vi "SMO_Query.vi"(0 "System no.":i32=1 min=1 max=4 step=1, 2 "Axes to query":string[](array[string]), 3 "All axes?":bool, 4 "Axis identifier?":bool=TRUE, 5 "error in":errorcluster) -> (14 "Current motor output":dbl[](array[numeric]) format="%.6f", 19 "error out":errorcluster)   [LabVIEW 2020]
doc: "Returns the current motor output. In servo-on mode, the actual value as set by the regulator is reported. In servo-off mode, the value set by the last SMO command is reported.\n\nC-702, C-848, C-865, C-866, C-867, C-877, C-880, C-884, C-891, E-871, Hydra, Mercury_GCS: If All axes? = TRUE, then Axis identifier? can be FALSE\n\nC-843, C-843.PM, C-844: If All axes? = TRUE, then Axis identifier? must be TRUE\n\nE-873: If All axes? = TRUE, then Axis identifier? can be FALSE."
panel:
  # "Returns the current motor output. In servo-on mode, the actual value\nas set by the regulator is reported. In servo-off mode, the value set by\nthe last SMO command is reported."
  # "If all axes: use"
  # "Query"
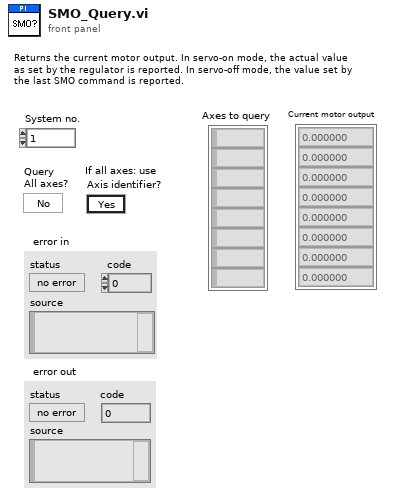
[diagram p1: front panel]
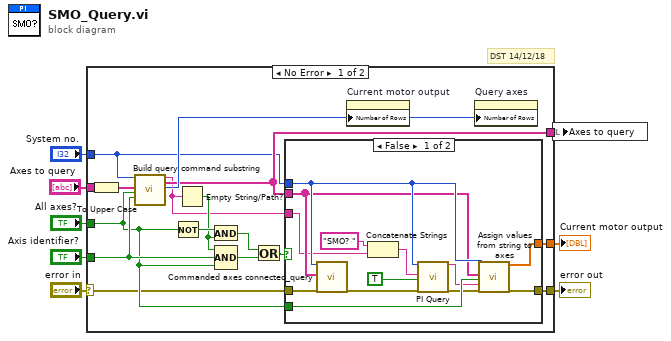
[diagram p0: block diagram]
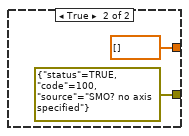
[diagram p2: hidden frame]
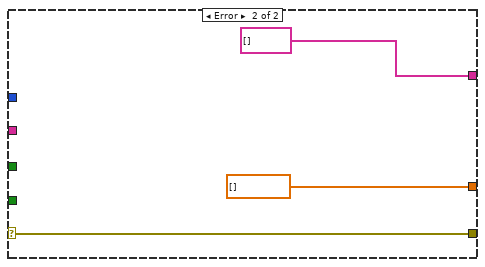
[diagram p3: hidden frame]
diagram:
  # "DST 14/12/18"
  n1 = case shown="No Error" "error in" {
    selector: "error in" -> [w10 w40]
    tunnel: [w24 dbl[] [] ("Values")] -> w8
    tunnel: "Axes to query" -> [w23 _]
    tunnel: [w22 w40] -> w6
    tunnel: "System no." -> [w9 _]
    tunnel: [w19 string[] [] ("Axes to query out")] -> w4
    tunnel: "Axis identifier?" -> [w16 _]
    tunnel: "All axes?" -> [w15 _]
    frame No Error {
      n2 = To Upper Case(1:w23) -> (0:w21:string[])
      n3 = call "Build query command substring.vi"("System no."=w9, "Axes to query in"=w21, "Query\nAll axes?"=w15, "For all axes: use\nAxis identifier?"=w16) -> ("Command substring"=w12:string, "Axes to query out"=w19:string[], "Number of rows"=w20:u32)  [unwired: 2 in, 11 out]
      n4 = Not(x=w15) -> (.not. x?=w18:bool)
      n5 = Empty String/Path?(string/path=w12) -> (empty?=w13:bool)
      n6 = And(x=w18, y=w13) -> (x .and. y?=w17:bool)
      n7 = Compound Arithmetic op=AND(w13, w16, w15) -> (w14:bool)
      n8 = Or(x=w17, y=w14) -> (x .or. y?=w11:bool)
      n9 = case shown="False" w11 {
        tunnel: [w34 dbl[] [] ("Values")] -> w24
        tunnel: w10 -> [w33 _]
        tunnel: [w30 errorcluster {"status"=TRUE, "code"=100, "source"="SMO? no axis specified"} ("error out")] -> w22
        tunnel: w9 -> [w32 _]
        tunnel: w19 -> [w31 _]
        tunnel: w15 -> [w29 _]
        tunnel: w12 -> [w27 _]
        frame False {
          n10 = call "Commanded axes connected_query.vi"("System no."=w32, "Commanded axes"=w31, "error in"=w33) -> ("error out"=w28:errorcluster)  [unwired: 1 in, 15 out]
          n11 = Concatenate Strings("SMO? ", w27) -> (w35:string)
          n12 = call "PI Query.vi"("System no."=w32, "String to send"=w35, "Attach termination char.?"=TRUE ("Attach Linefeed?"), "error in"=w28) -> ("String read"=w26:string, "error out"=w25:errorcluster)  [unwired: 3 in, 11 out]
          n13 = call "Assign values from string to axes.vi"("System no."=w32, "Queried axes"=w31, "All axes queried?"=w29, "Input String"=w26, "error in"=w25) -> ("Values"=w34:dbl[], "error out"=w30:errorcluster)  [unwired: 4 in, 9 out]
        }
        frame True {
        }
      }
      n14 = property on="Current motor output" class="Arr (strict)"("Number of Rows"=w20) -> ()  [unwired: 2 in, 2 out]
      n15 = property on="Query axes" class="Arr (strict)"("Number of Rows"=w20) -> ()  [unwired: 2 in, 2 out]
    }
    frame Error {
    }
  }
  "error out" <- w6
  "Current motor output" <- w8
  n16 = local write "Axes to query"(w4) -> ()
